vi "例4-8.vi"() -> ()   [LabVIEW 2019]
panel:
  in  "确定按钮":bool
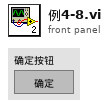
[diagram p1: front panel]
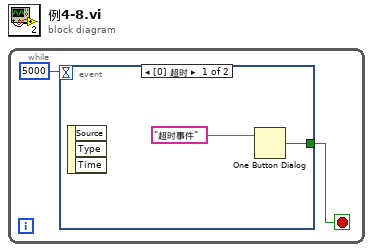
[diagram p0: block diagram]
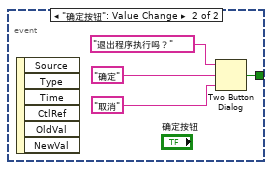
[diagram p2: hidden frame]
diagram:
  n1 = while {
    stop <- w1 stop-if-true
    n2 = event shown="[0] 超时" {
      selector: _ -> [_ _]
      dyn-events: _ -> [_ _]
      timeout: 5000 -> [_ _]
      tunnel: [w3 w5] -> w1
      event Timeout {
        n3 = event-data() -> ()  [unwired: 1 in, 3 out]
        n4 = One Button Dialog(message="超时事件" ("消息")) -> (true=w3:bool)  [unwired: 1 in]
      }
      event "确定按钮": Value Change {
        n5 = event-data() -> ()  [unwired: 1 in, 6 out]
        n6 = Two Button Dialog(message="退出程序执行吗？", 1:"取消", 2:"确定") -> (T button?=w5:bool)
      }
    }
  }
